vi "Read Deps.vi"(11 "ProjectItem in":refnum<class "ProjectItem.lvclass">) -> (2 "Deps":set{string}(c389), 3 "ProjectItem out":refnum<class "ProjectItem.lvclass">)   [LabVIEW 2019, in "SolutionBuilder.lvlib" / "ProjectItem.lvclass"]
uses:
  ProjectItem.lvclass
  ProjectItem.lvclass/ProjectItem.ctl
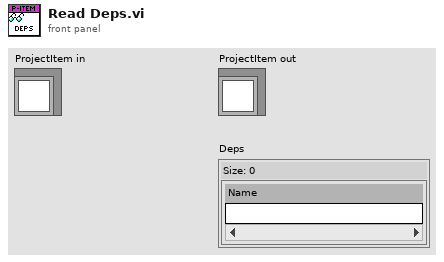
[diagram p1: front panel]
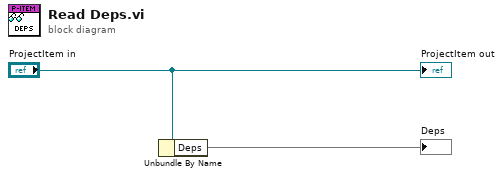
[diagram p0: block diagram]
diagram:
  n1 = Unbundle By Name("ProjectItem in") -> ("Deps"=→"Deps":set{string})
  "ProjectItem out" <- "ProjectItem in"
